vi "SOFandEOF_del.vi"(8 "error in (no error)":errorcluster, 11 "ISO 14443 A DOWN in":refnum<class "ISO 14443 A DOWN.lvclass">) -> (0 "error out":errorcluster, 3 "ISO 14443 A DOWN out":refnum<class "ISO 14443 A DOWN.lvclass">)   [LabVIEW 2019, in "ISO 14443 A DOWN.lvclass"]
uses:
  ISO 14443 A DOWN.lvclass
  TypeDef/Store.ctl
  ISO 14443 A DOWN.lvclass/ISO 14443 A DOWN.ctl
  RFID system.lvclass
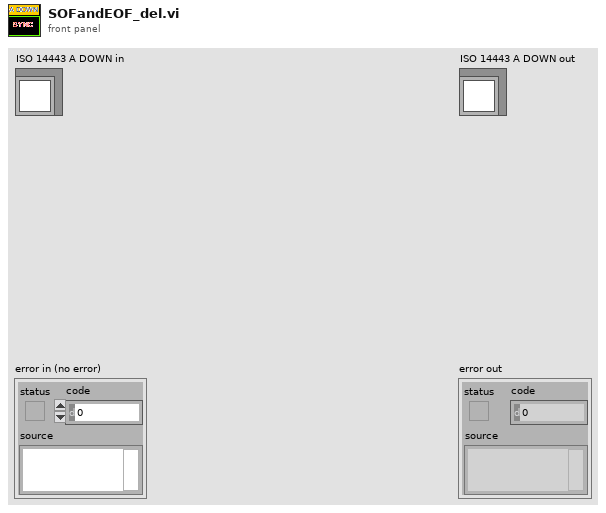
[diagram p1: front panel]
types:
  T1 = typedef "Store.ctl" = enum16{"envelope", "noise", "demSubCar", "CH_frame", "Decode", "demodulate", "in", "out", "sum", "subCarrier", "frame", "command", "encode", "modulate", "encode_UP", "modulate_up", "demod_up", "envelop_up", "sum_up", "out_up", "in_up"}
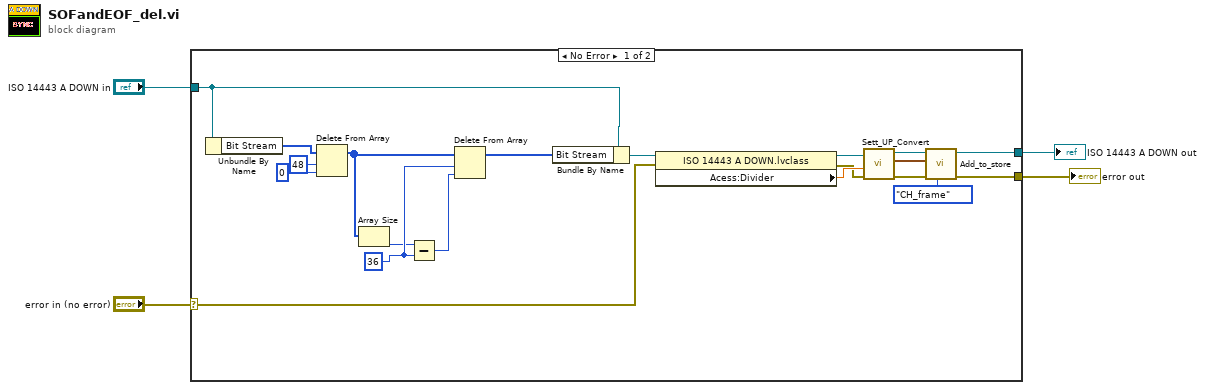
[diagram p0: block diagram]
diagram:
  n1 = case shown="No Error" "error in (no error)" {
    selector: "error in (no error)" -> [w7 w25]
    tunnel: "ISO 14443 A DOWN in" -> [w17 w26]
    tunnel: [w14 w26] -> w3
    tunnel: [w12 w25] -> w1
    frame No Error {
      w22 = 36 ("length")
      n2 = Unbundle By Name(w17) -> ("Bit Stream"=w18:u8[])
      n3 = Delete From Array(array=w18, length=48, index=0) -> (array with subset deleted=w24:u8[])  [unwired: 1 out]
      n4 = Array Size(array=w24) -> (size(s)=w20:i32)
      n5 = Subtract(x=w20, y=w22) -> (x-y=w21:i32)
      n6 = Delete From Array(array=w24, length=w22, index=w21) -> (array with subset deleted=w5:u8[])  [unwired: 1 out]
      n7 = Bundle By Name(cluster=w17, "Bit Stream"=w5) -> (w16:refnum<class "ISO 14443 A DOWN.lvclass">)
      n8 = property class="ISO 14443 A DOWN.lvclass"(reference=w16, error in=w7) -> (reference out=w9:refnum<class "ISO 14443 A DOWN.lvclass">, error out=w6:errorcluster, "Acess:Divider"=w8:dbl)
      n9 = call-dynamic "Sett_UP_Convert.vi"("error in (no error)"=w6, "Divider(1)"=w8, "ISO 14443 A DOWN in"=w9) -> ("error out"=w13:errorcluster, "Waveform"=w10:waveform(dbl), "ISO 14443 A DOWN out"=w15:refnum<class "ISO 14443 A DOWN.lvclass">)  [unwired: 6 in]
      n10 = call "Add_to_store.vi"("Store"=Store."CH_frame", "error in (no error)"=w13, "Waveform"=w10, "RFID system in"=w15) -> ("error out"=w12:errorcluster, "RFID system out"=w14:refnum<class "ISO 14443 A DOWN.lvclass">)  [unwired: 6 in]
    }
    frame Error {
    }
  }
  "error out" <- w1
  "ISO 14443 A DOWN out" <- w3
